vi "Addr to Index.vi"(10 "addr":i32, 11 "RRAM Mode":u16) -> (3 "index":i32)   [LabVIEW 2018]
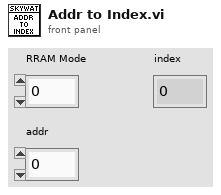
[diagram p1: front panel]
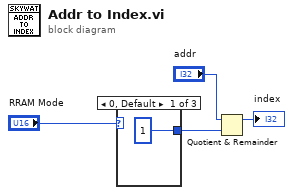
[diagram p0: block diagram]
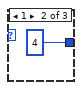
[diagram p2: hidden frame]
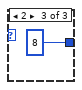
[diagram p3: hidden frame]
diagram:
  n1 = case shown="0, Default" "RRAM Mode" {
    tunnel: [1 4 8] -> w3
    frame 0, Default {
    }
    frame 1 {
    }
    frame 2 {
    }
  }
  n2 = Quotient & Remainder(x="addr", y=w3) -> (x-y*floor(x/y)=→"index":i32)  [unwired: 1 out]
